vi "Transform.vi"(4 "P":T1={"x (cm)"=1.0, "y (cm)"=-3.0, "z (cm)"=1.0} {"x (cm)" format="%.2f"; "z (cm)" format="%.2f"; "y (cm)" format="%.2f"}) -> (2 "transfrom matrix":dbl[][](array[numeric]) format="%.2f")   [LabVIEW 2022 SP3]
uses:
  <vilib>/Analysis/baseanly.llb/Real A x B.vi
  <vilib>/Analysis/NI_AALPro.lvlib
  <vilib>/Analysis/NI_AALBase.lvlib
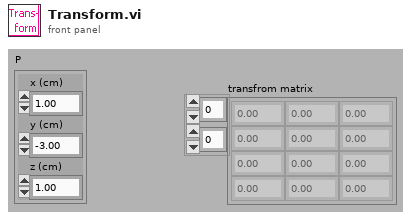
[diagram p1: front panel]
types:
  T1 = cluster{"x (cm)":dbl, "y (cm)":dbl, "z (cm)":dbl}
  T2 = typedef "NI_Matrix.lvlib/RealMatrix.ctl" = dbl[][]
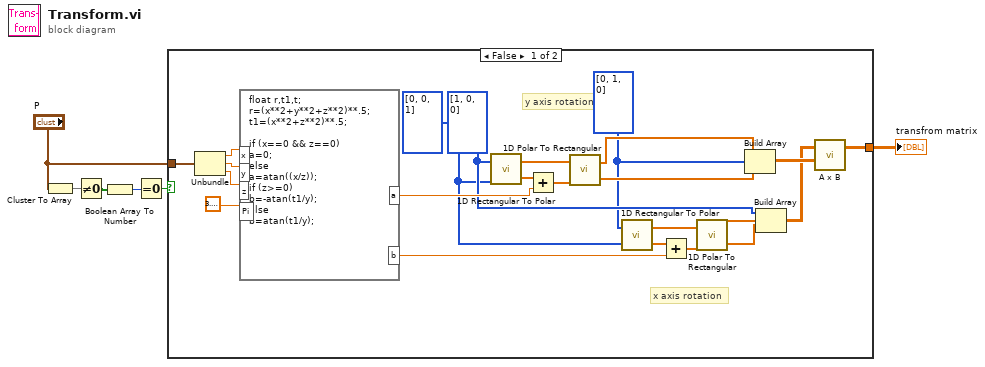
[diagram p0: block diagram]
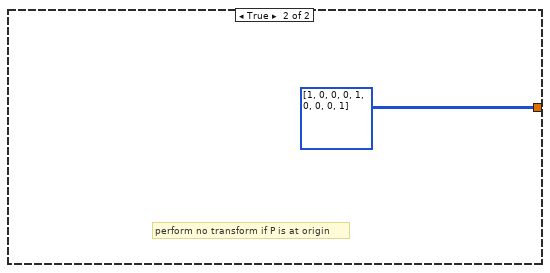
[diagram p2: hidden frame]
diagram:
  n1 = Cluster To Array(cluster="P") -> (array=w4:dbl[])
  n2 = Not Equal To 0?(x=w4) -> (x != 0?=w3:bool[])
  n3 = Boolean Array To Number(Boolean array=w3) -> (number=w2:u32)
  n4 = Equal To 0?(x=w2) -> (x = 0?=w1:bool)
  n5 = case shown="False" w1 {
    tunnel: "P" -> [w8 _]
    tunnel: [w7 i32[][] [[1, 0, 0], [0, 1, 0], [0, 0, 1]] ("A x Vector 2")] -> w6
    frame False {
      w13 = i32[] [0, 1, 0] ("A x Vector 2")
      w14 = i32[] [0, 0, 1] ("A x Vector 2")
      w17 = i32[] [1, 0, 0] ("A x Vector 2")
      # "x axis rotation"
      # "y axis rotation"
      n6 = Unbundle(w8) -> ("x (cm)"=w27:dbl, "y (cm)"=w26:dbl, "z (cm)"=w29:dbl)
      n7 = formula code="float r,t1,t;\nr=(x**2+y**2+z**2)**.5;\nt1=(x**2+z**2)**.5;\n\nif (x==0 && z==0)\na=0;\nelse\na=atan((x/z));\nif (z>=0)\nb=-atan(t1/y);\nelse\nb=atan(t1/y);"("x"=w27, "y"=w26, "z"=w29, "Pi"=3.141592653589793) -> ("a"=w23:dbl, "b"=w18:dbl)
      n8 = call <vilib>:"1D Rectangular To Polar.vi"("X"=w17, "Y"=w14) -> ("Magnitude"=w16:dbl[], "Phase"=w25:dbl[])  [unwired: 1 out]
      n9 = Add(x=w25, y=w23) -> (x+y=w24:dbl[])
      n10 = call <vilib>:"1D Polar To Rectangular.vi"("Magnitude"=w16, "Phase"=w24) -> ("X"=w15:dbl[], "Y"=w22:dbl[])  [unwired: 1 out]
      n11 = call <vilib>:"1D Rectangular To Polar.vi"("X"=w13, "Y"=w14) -> ("Magnitude"=w19:dbl[], "Phase"=w21:dbl[])  [unwired: 1 out]
      n12 = Add(x=w21, y=w18) -> (x+y=w20:dbl[])
      n13 = call <vilib>:"1D Polar To Rectangular.vi"("Magnitude"=w19, "Phase"=w20) -> ("X"=w12:dbl[], "Y"=w11:dbl[])  [unwired: 1 out]
      n14 = Build Array(w15, w13, w22) -> (w10:dbl[][])
      n15 = Build Array(w17, w12, w11) -> (w9:dbl[][])
      n16 = call-poly <vilib>:"A x B.vi"("B"=w10, "A"=w9) -> ("A x B"=w7:T2)  [unwired: 1 out]
    }
    frame True {
      # "perform no transform if P is at origin"
    }
  }
  "transfrom matrix" <- w6
